vi "LooseVI.vi"(8 "Numeric":dbl=4.0) -> (0 "Numeric 2":dbl)   [LabVIEW 2022 SP3]
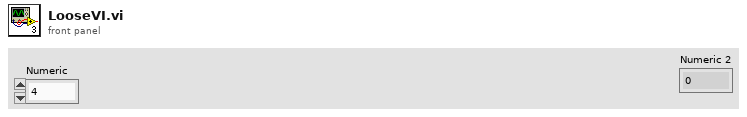
[diagram p1: front panel]
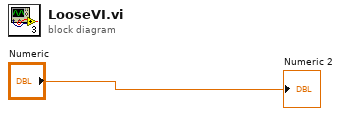
[diagram p0: block diagram]
diagram:
  "Numeric 2" <- "Numeric"
